vi "AlliGator Load SS2 FLI Dataset Prelude.vi"(8 "error in (no error)":errorcluster, 11 "File Path in":path) -> (0 "error out":errorcluster, 1 "Metadata":string, 2 "FLI Data File Information":T1, 3 "File Path out":path, 4 "Data Description":string)   [LabVIEW 2021, in "AlliGator Files.lvlib"]
doc: "Preliminary steps to loading a SS2 dataset."
uses:
  AlliGator Files.lvlib
  AlliGator FLI Data File Information.ctl
  Phasor/Phasor Fluorescence Lifetime Parameters v3.ctl
  AlliGator FLI Dataset Type.ctl
  AlliGator HDF5.lvlib
  Phasor/Phasor.lvlib
panel:
  # "see the AlliGator License on the block diagram (Ctrl+E or Window:Show Block Diagram)"
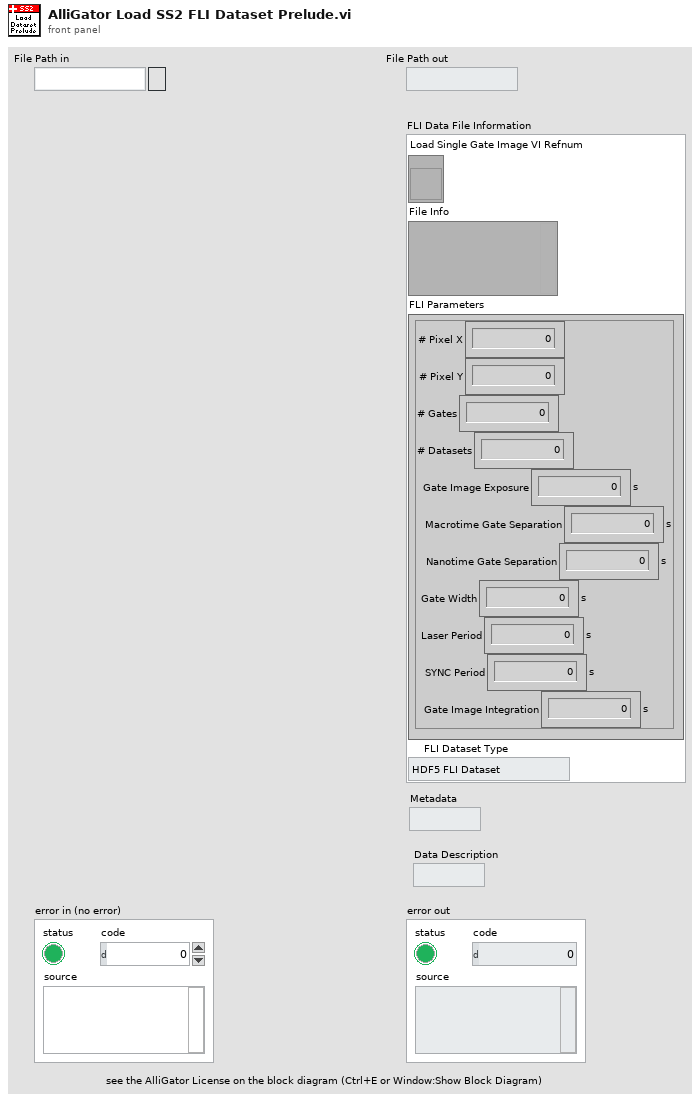
[diagram p1: front panel]
types:
  T1 = typedef "AlliGator HDF5.lvlib/AlliGator FLI Data File Information.ctl" = cluster{"Load Single Gate Image VI Refnum":refnum<vi>, "File Info":variant, "FLI Parameters":T2, "FLI Dataset Type":T3}
  T2 = typedef "Phasor.lvlib/Phasor Fluorescence Lifetime Parameters v3.ctl" = cluster{"# Pixel X":i32, "# Pixel Y":i32, "# Gates":i32, "# Datasets":i32, "Gate Image Exposure":dbl[unit], "Macrotime Gate Separation":dbl[unit], "Nanotime Gate Separation":dbl[unit], "Gate Width":dbl[unit], "Laser Period":dbl[unit], "SYNC Period":dbl[unit], "Gate Image Integration":dbl[unit]}
  T3 = typedef "AlliGator Files.lvlib/AlliGator FLI Dataset Type.ctl" = enum16{"HDF5 FLI Dataset", "Gate Image Folder", ".sdt FLI Dataset (Becker & Hickl)", ".ptu FLI Dataset (PicoQuant)", "SS1 FLI Dataset", "SS2 FLI Dataset", "I/m/phi Dataset", ".bin FLI Dataset (PicoQuant Binned)", ".bin FLI Dataset (Piccolo Binned)"}
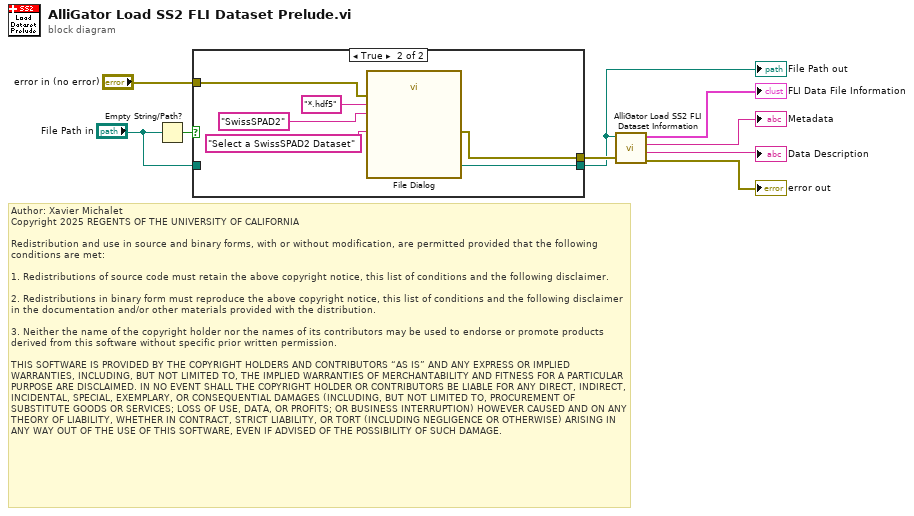
[diagram p0: block diagram]
diagram:
  # "Author: Xavier Michalet\nCopyright 2025 REGENTS OF THE UNIVERSITY OF CALIFORNIA\n\nRedistribution and use in source and binary forms, with or without modification, are permitted provided that the following conditions are met:\n\n1. Redistributions of source code must retain the above copyright notice, this list of conditions and the following disclaimer.\n\n2. Redistributions in binary form must reproduce the above copyright notice, this list of conditions and the following disclaimer in the documentation and/or other materials provided with the distribution.\n\n3. Neither the name of the copyright holder nor the names of its contributors may be used to endorse or promote products derived from this software without specific prior written permission.\n\nTHIS SOFTWARE IS PROVIDED BY THE COPYRIGHT HOLDERS AND CONTRIBUTORS “AS IS” AND ANY EXPRESS OR IMPLIED WARRANTIES, INCLUDING, BUT NOT LIMITED TO, THE IMPLIED WARRANTIES OF MERCHANTABILITY AND FITNESS FOR A PARTICULAR PURPOSE ARE DISCLAIMED. IN NO EVENT SHALL THE COPYRIGHT HOLDER OR CONTRIBUTORS BE LIABLE FOR ANY DIRECT, INDIRECT, INCIDENTAL, SPECIAL, EXEMPLARY, OR CONSEQUENTIAL DAMAGES (INCLUDING, BUT NOT LIMITED TO, PROCUREMENT OF SUBSTITUTE GOODS OR SERVICES; LOSS OF USE, DATA, OR PROFITS; OR BUSINESS INTERRUPTION) HOWEVER CAUSED AND ON ANY THEORY OF LIABILITY, WHETHER IN CONTRACT, STRICT LIABILITY, OR TORT (INCLUDING NEGLIGENCE OR OTHERWISE) ARISING IN ANY WAY OUT OF THE USE OF THIS SOFTWARE, EVEN IF ADVISED OF THE POSSIBILITY OF SUCH DAMAGE."
  n1 = Empty String/Path?(string/path="File Path in") -> (empty?=w1:bool)
  n2 = case shown="True" w1 {
    tunnel: "error in (no error)" -> [w10 w17]
    tunnel: [w11 w16] -> w4
    tunnel: [w10 w15] -> w5
    tunnel: "File Path in" -> [w11 _]
    frame False {
    }
    frame True {
      n3 = call "File Dialog"("prompt"="Select a SwissSPAD2 Dataset", "error in"=w17, "pattern (all files)"="*.hdf5", "pattern label"="SwissSPAD2") -> ("selected path"=w16:path, "error out"=w15:errorcluster)  [unwired: 8 in, 2 out]
    }
  }
  "File Path out" <- w4
  n4 = call "AlliGator Load SS2 FLI Dataset Information.vi"("error in (no error)"=w5, "Image Folder"=w4) -> ("error out"=→"error out":errorcluster, "Data Description"=→"Data Description":string, "Metadata"=→"Metadata":string, "FLI Data File Information"=→"FLI Data File Information":T1)  [unwired: 6 in]
